vi "Global 1.vi"() -> ()   [LabVIEW 2015]
panel:
  out "BLE Set Packet (data)":u8[][](array[numeric])
  out "BLE Set Packet (buf)":u8[](array[numeric])
  out "BLE Set Packet":bool=TRUE
  out "BLE Mon Packet (data)":u8[][](array[numeric])
  out "BLE Mon Packet (buf)":u8[](array[numeric])
  out "BLE Mon Packet":bool=TRUE
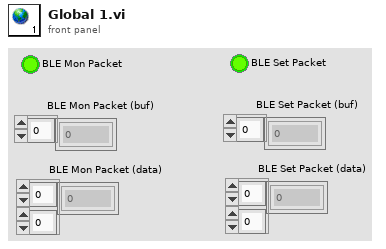
[diagram p1: front panel]
diagram:
